vi "ini_build_objects_list_recoursive.vi"(6 "base cluster":string, 8 "error in":errorcluster, 9 "owning vi rel path":string, 10 "owner chain (empty)":string, 11 "Ctl Refnum":refnum<vi>) -> (0 "error out":errorcluster, 3 "item":string)   [LabVIEW 2020]
uses:
  <vilib>/regexp/Match Regular Expression.xnode
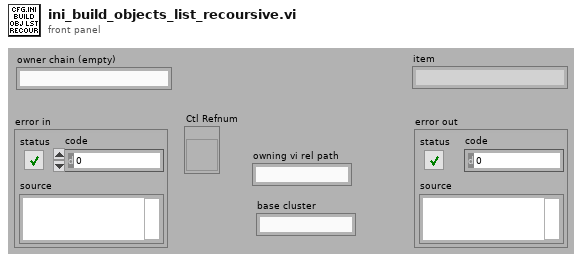
[diagram p1: front panel]
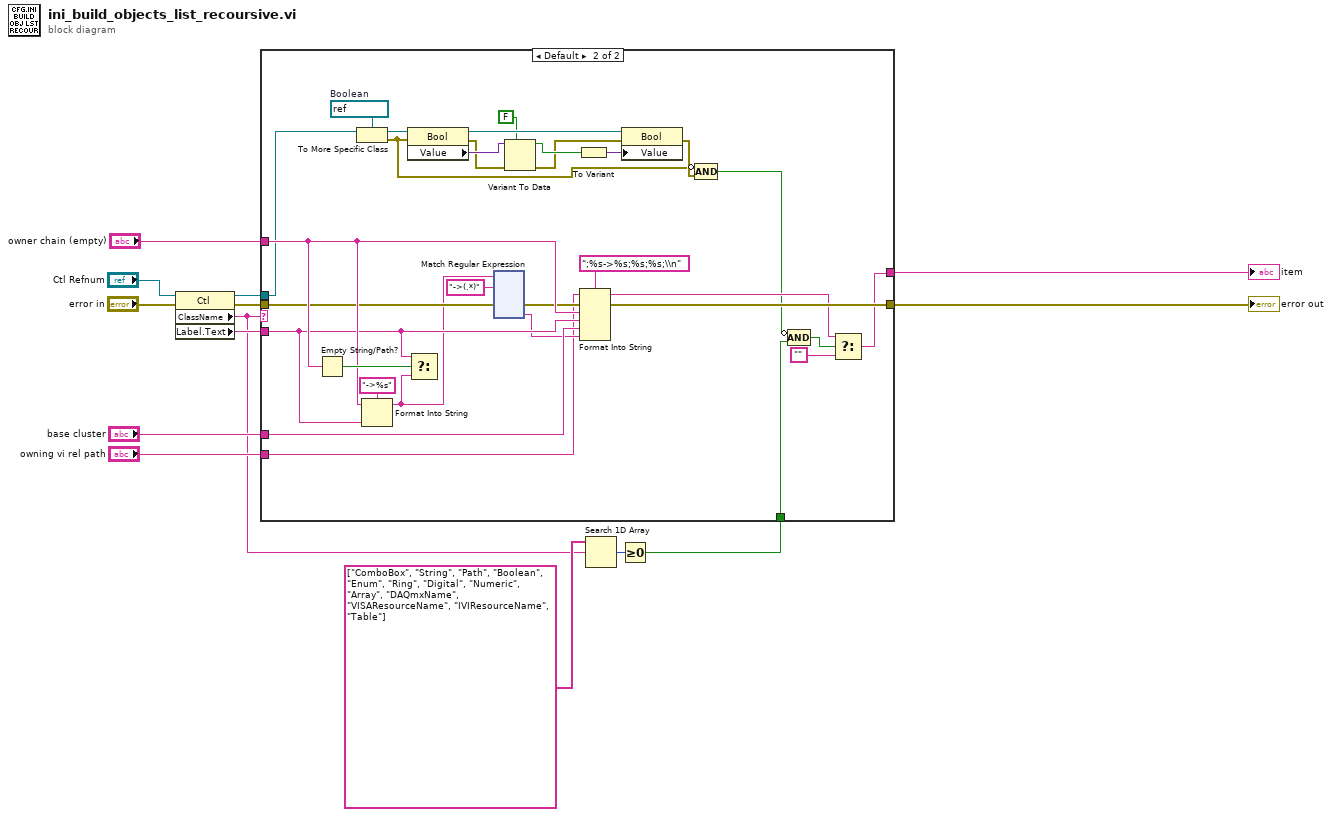
[diagram p0: block diagram]
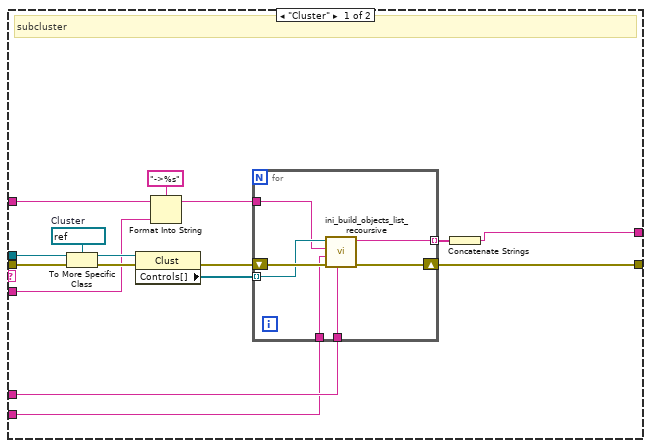
[diagram p2: hidden frame]
diagram:
  n1 = property class="Ctl"(reference="Ctl Refnum", error in="error in") -> (reference out=w1:refnum<vi>, error out=w11:errorcluster, "ClassName"=w2:string, "Label.Text"=w8:string)
  n2 = Search 1D Array(1D array=string[] ["ComboBox", "String", "Path", "Boolean", "Enum", "Ring", "Digital", "Numeric", "Array", "DAQmxName", "VISAResourceName", "IVIResourceName", "Table"], element=w2) -> (index of element=w6:i32)  [unwired: 1 in]
  n3 = Greater Or Equal To 0?(x=w6) -> (x >= 0?=w4:bool)
  n4 = case shown="Default" w2 {
    tunnel: w1 -> [w30 w39]
    tunnel: w11 -> [w28 w62]
    tunnel: "owner chain (empty)" -> [w19 w64]
    tunnel: [w22 w55] -> w5
    tunnel: [w21 w67] -> w12
    tunnel: "base cluster" -> [w20 w66]
    tunnel: w8 -> [w16 w63]
    tunnel: w4 -> [_ w52]
    tunnel: "owning vi rel path" -> [w15 w53]
    frame "Cluster" {
      w29 = refnum<vi> refnum  # Cluster
      # "subcluster"
      n5 = To More Specific Class(target class=w29, reference=w30, error in=w28) -> (specific class reference=w26:refnum<vi>, error out=w27:errorcluster)
      n6 = property class="Clust"(reference=w26, error in=w27) -> (error out=w24:errorcluster, "Controls[]"=w25:refnum<vi>[])  [unwired: 1 out]
      n7 = Format Into String(format string="->%s", initial string=w19, w16) -> (resulting string=w17:string)  [unwired: 1 in, 1 out]
      n8 = for {
        tunnel: w25 -> [w36] mode=indexing
        tunnel: w17 -> [w33]
        shift-right: [w35] -> w21
        shift-left: w24 -> [w37]
        tunnel: [w32] -> w23 mode=indexing
        tunnel: w20 -> [w34]
        tunnel: w15 -> [w31]
        n9 = call "ini_build_objects_list_recoursive.vi"("base cluster"=w34, "error in"=w37, "owning vi rel path"=w31, "owner chain (empty)"=w33, "Ctl Refnum"=w36) -> ("error out"=w35:errorcluster, "item"=w32:string)  [unwired: 5 in]
      }
      n10 = Concatenate Strings(w23) -> (w22:string)
    }
    frame Default {
      w49 = refnum<vi> refnum  # Boolean
      n11 = Empty String/Path?(string/path=w64) -> (empty?=w65:bool)
      n12 = To More Specific Class(target class=w49, reference=w39) -> (specific class reference=w50:refnum<vi>, error out=w44:errorcluster)  [unwired: 1 in]
      n13 = Format Into String(format string="->%s", initial string=w64, w63) -> (resulting string=w58:string)  [unwired: 1 in, 1 out]
      n14 = property class="Bool"(reference=w50, error in=w44) -> (reference out=w48:refnum<vi>, error out=w40:errorcluster, "Value"=w46:variant)
      n15 = Select(t=w63, s=w65, f=w58) -> ()  [unwired: 1 out]
      n16 = xnode "Match Regular Expression"("input string"=w58, "regular expression"="->(.*)", "error in"=w62) -> ("error out"=w61:errorcluster, "submatch 1"=w59:string)  [unwired: 3 in, 4 out]
      n17 = Variant To Data(error in=w40, type=FALSE, Variant=w46) -> (data=w45:bool, error out=w43:errorcluster)
      n18 = To Variant(anything=w45) -> (Variant=w41:variant)
      n19 = Format Into String(format string=";%s->%s;%s;%s;\\n", initial string=w53, error in=w61, w64, w63, w66, w59) -> (resulting string=w56:string, error out=w67:errorcluster)
      n20 = property class="Bool"(reference=w48, error in=w43, "Value"=w41) -> (error out=w47:errorcluster)  [unwired: 1 out]
      n21 = Compound Arithmetic op=AND(invert w44, w47) -> (w38:bool)
      n22 = Compound Arithmetic op=AND(invert w38, w52) -> (w51:bool)
      n23 = Select(t=w56, s=w51, f="") -> (s? t:f=w55:string)
    }
  }
  "error out" <- w12
  "item" <- w5
